vi "generate reference signal.vi"(8 "error in (no error)":errorcluster, 11 "Dynamic-System in":refnum<class "Dynamic-System.lvclass">) -> (0 "error out":errorcluster, 2 "Reference Array":cluster{"Time":dbl[], "Reference":dbl[]}, 3 "Dynamic-System out":refnum<class "Dynamic-System.lvclass">)   [LabVIEW 2025, in "Dynamic-System.lvclass"]
uses:
  Dynamic-System.lvclass
  Dynamic-System.lvclass/Dynamic-System.ctl
panel:
  out "Reference":dbl[](array[numeric])
  out "Time":dbl[](array[numeric])
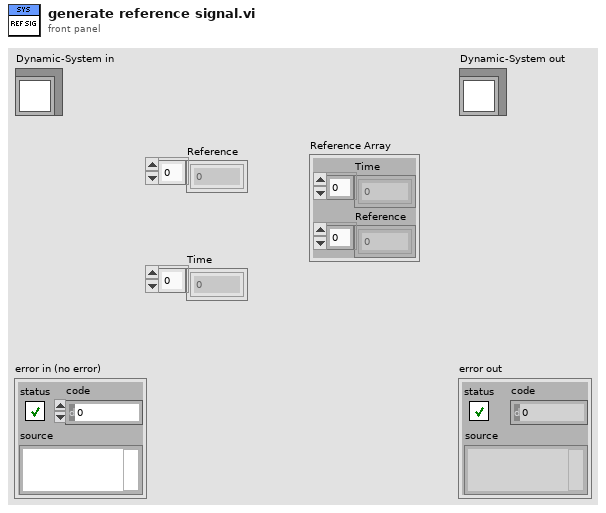
[diagram p1: front panel]
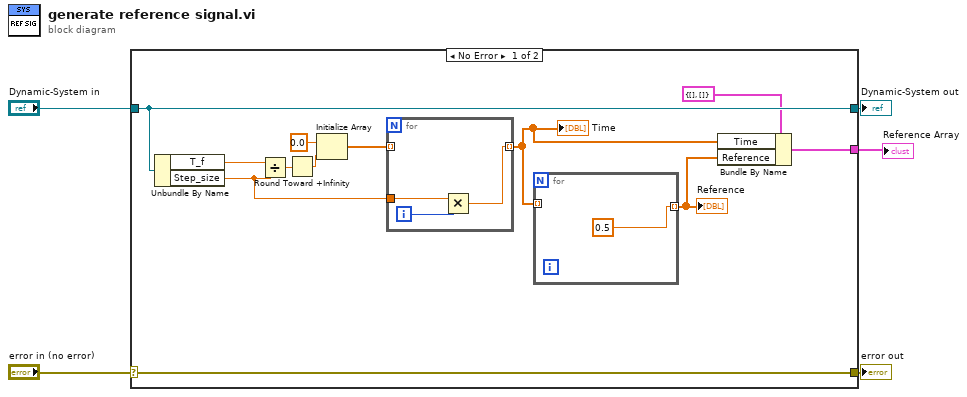
[diagram p0: block diagram]
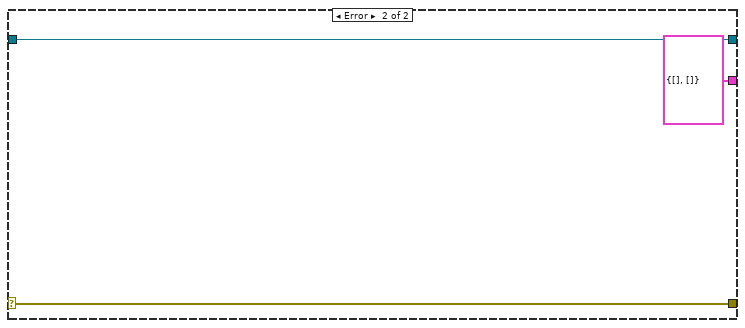
[diagram p2: hidden frame]
diagram:
  n1 = case shown="No Error" "error in (no error)" {
    selector: "error in (no error)" -> [w17 w24]
    tunnel: [w17 w24] -> w4
    tunnel: [w16 w23] -> w2
    tunnel: "Dynamic-System in" -> [w16 w23]
    tunnel: [w8 cluster{"Time":dbl[], "Reference":dbl[]} {"Time"=[], "Reference"=[]} ("cluster")] -> w1
    frame No Error {
      n2 = Unbundle By Name(w16) -> ("T_f"=w15:dbl, "Step_size"=w12:dbl)
      n3 = Divide(x=w15, y=w12) -> (x/y=w7:dbl)
      n4 = Round Toward +Infinity(x=w7) -> (ceil(x): smallest int >= x=w6:dbl)
      n5 = Initialize Array(0.0 ("element"), w6) -> (w13:dbl[])
      n6 = for {
        tunnel: w13 -> [_] mode=indexing
        tunnel: w12 -> [w20]
        tunnel: [w19] -> w10 mode=indexing
        i -> [w21]
        n7 = Multiply(x=w20, y=w21) -> (x*y=w19:dbl)
      }
      "Time" <- w10
      n8 = for {
        tunnel: w10 -> [_] mode=indexing
        tunnel: [0.5] -> w9 mode=indexing
      }
      "Reference" <- w9
      n9 = Bundle By Name(cluster=cluster{"Time":dbl[], "Reference":dbl[]} {"Time"=[], "Reference"=[]}, "Time"=w10, "Reference"=w9) -> (w8:cluster{"Time":dbl[], "Reference":dbl[]})
    }
    frame Error {
    }
  }
  "error out" <- w4
  "Dynamic-System out" <- w2
  "Reference Array" <- w1
